vi "optimize.vi"(5 "learning_rate":dbl=0.01, 6 "num_iterations":i32=500, 7 "Y":dbl[][](array[numeric]), 8 "X":dbl[][](array[numeric]), 9 "b":dbl, 10 "w":dbl[][](array[numeric])) -> (0 "dw":dbl[][](array[numeric]), 1 "db":dbl, 2 "trained_b":dbl, 3 "trained_W":dbl[][](array[numeric]), 4 "costs":dbl[](array[numeric]))   [LabVIEW 2020]
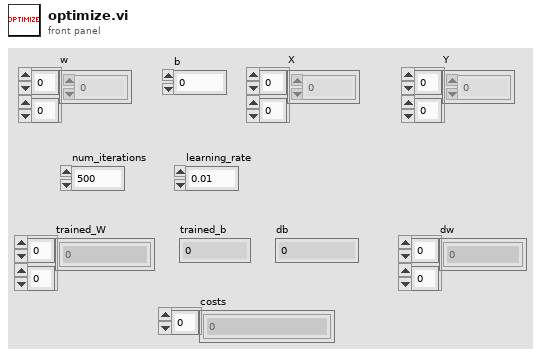
[diagram p1: front panel]
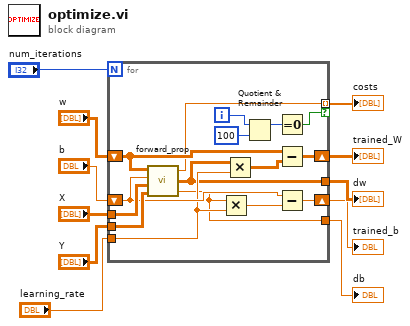
[diagram p0: block diagram]
diagram:
  n1 = for {
    N: "num_iterations" -> [_]
    tunnel: "X" -> [w27]
    tunnel: "Y" -> [w26]
    tunnel: "learning_rate" -> [w20]
    shift-right: [w23] -> w3
    shift-left: "w" -> [w25]
    shift-right: [w19] -> w2
    shift-left: "b" -> [w22]
    tunnel: [w15] -> w1 mode=indexing if=w14
    tunnel: [w13] -> w5
    tunnel: [w12] -> w4
    i -> [w18]
    n2 = call "forward_prop.vi"("Y"=w26, "X"=w27, "b"=w22, "W"=w25) -> ("db"=w12:dbl, "dw"=w13:dbl[][], "cost"=w15:dbl)
    n3 = Multiply(x=w12, y=w20) -> (x*y=w21:dbl)
    n4 = Multiply(x=w13, y=w20) -> (x*y=w24:dbl[][])
    n5 = Quotient & Remainder(x=w18, y=100) -> (x-y*floor(x/y)=w16:i32)  [unwired: 1 out]
    n6 = Equal To 0?(x=w16) -> (x = 0?=w14:bool)
    n7 = Subtract(x=w25, y=w24) -> (x-y=w23:dbl[][])
    n8 = Subtract(x=w22, y=w21) -> (x-y=w19:dbl)
  }
  "dw" <- w5
  "db" <- w4
  "trained_W" <- w3
  "trained_b" <- w2
  "costs" <- w1
